vi "Resolve.vi"(8 "error in (no error)":errorcluster, 10 "Result (None)":refnum<class>, 11 "Promise in":refnum<class "Promise.lvclass">) -> (0 "error out":errorcluster, 3 "Promise out":refnum<class "Promise.lvclass">)   [LabVIEW 2020, in "Promises.lvlib" / "Promise.lvclass"]
doc: "<b>THIS VI DOES NOT PROPAGATE ERRORS</b>\nThis VI will generate an error if the Promise has already been resolved or is otherwise invalid.\n\nResolves the Promise with the provided Result value unless an error is passed in which will be encapsulated into the response and sent to the Future to return."
uses:
  Promise.lvclass
  Promise.lvclass/Promise.ctl
  Result.ctl
  Result State.ctl
  Error Result/Error Result.lvclass/Error Result.ctl
  Variant/Variant.lvclass
  Error Result/Error Result.lvclass
  Promises.lvlib
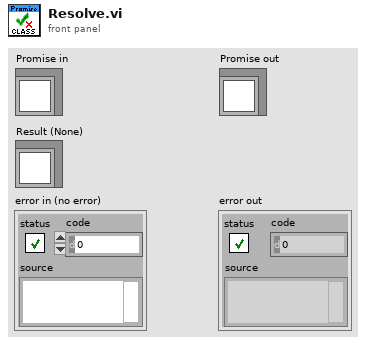
[diagram p1: front panel]
types:
  T1 = typedef "Promises.lvlib/Result.ctl" = cluster{"State":T2, "Value":refnum<class>}
  T2 = typedef "Promises.lvlib/Result State.ctl" = enum16{"Unset", "Error", "Success"}
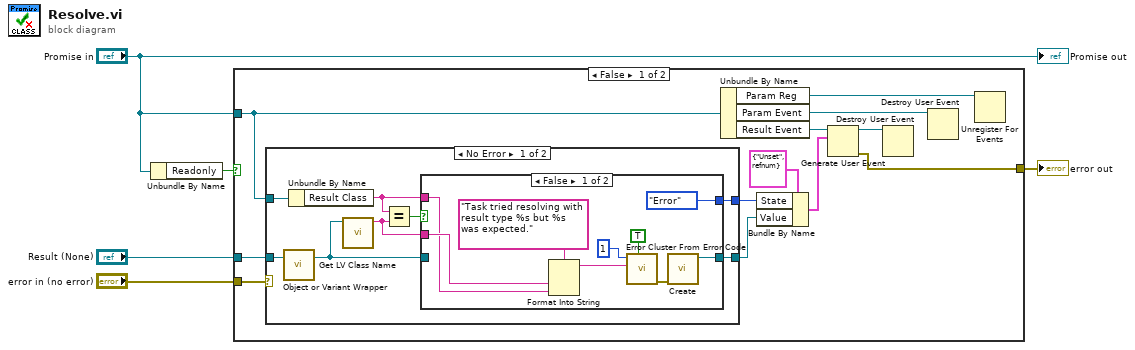
[diagram p0: block diagram]
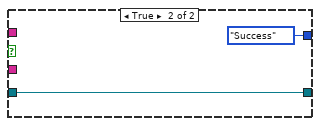
[diagram p2: hidden frame]
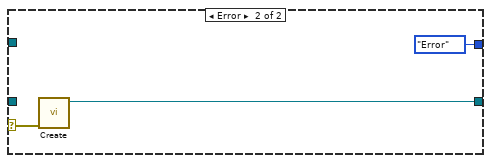
[diagram p3: hidden frame]
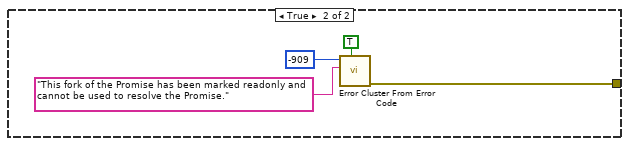
[diagram p4: hidden frame]
diagram:
  n1 = Unbundle By Name("Promise in") -> ("Readonly"=w1:bool)
  n2 = case shown="False" w1 {
    tunnel: "error in (no error)" -> [w17 _]
    tunnel: "Result (None)" -> [w16 _]
    tunnel: [w9 w43] -> w3
    tunnel: "Promise in" -> [w8 _]
    frame False {
      n3 = case shown="No Error" w17 {
        selector: w17 -> [_ w39]
        tunnel: w16 -> [w24 _]
        tunnel: [w20 w38] -> w13
        tunnel: w8 -> [w25 _]
        tunnel: [w19 Result_State."Error" ("Result State")] -> w14
        frame No Error {
          n4 = call "Object or Variant Wrapper.vi"("LabVIEW Object"=w24) -> ("Object or Variant Wrapper"=w18:refnum<class>)  [unwired: 6 in]
          n5 = Unbundle By Name(w25) -> ("Result Class"=w22:string)
          n6 = call <vilib>:"Get LV Class Name.vi"("object"=w18) -> ("class name"=w21:string)  [unwired: 9 in, 1 out]
          n7 = Equal?(x=w22, y=w21) -> (x = y?=w23:bool)
          n8 = case shown="False" w23 {
            tunnel: w18 -> [_ w36]
            tunnel: w22 -> [w33 _]
            tunnel: w21 -> [w34 _]
            tunnel: [w27 w36] -> w20
            tunnel: [Result_State."Error" ("Result State") Result_State."Success" ("Result State")] -> w19
            frame False {
              n9 = Format Into String(format string="Task tried resolving with result type %s but %s was expected.", w34, w33) -> (resulting string=w31:string)  [unwired: 2 in, 1 out]
              n10 = call <vilib>:"Error Cluster From Error Code.vi"("show call chain? (False)"=TRUE, "error message (\"\")"=w31, "error code (0)"=1) -> ("error out"=w28:errorcluster)  [unwired: 6 in]
              n11 = call "Create.vi"("error in (no error)"=w28) -> ("Error Result out"=w27:refnum<class "Error Result.lvclass">)  [unwired: 9 in, 1 out]
            }
            frame True {
            }
          }
        }
        frame Error {
          n12 = call "Create.vi"("error in (no error)"=w39) -> ("Error Result out"=w38:refnum<class "Error Result.lvclass">)  [unwired: 9 in, 1 out]
        }
      }
      n13 = Unbundle By Name(w8) -> ("Param Reg"=w6:refnum<event-registration>, "Param Event"=w7:refnum<user-event>, "Result Event"=w15:refnum<user-event>)
      n14 = Bundle By Name(cluster=T1 {"State"=enum."Unset", "Value"=refnum} ("event data"), "State"=w14, "Value"=w13) -> (w11:T1)
      n15 = Generate User Event(user event=w15, event data cluster=w11) -> (user event out=w10:refnum<user-event>, error out=w9:errorcluster)  [unwired: 2 in]
      n16 = Destroy User Event(user event=w10) -> ()  [unwired: 1 in, 1 out]
      n17 = Destroy User Event(user event=w7) -> ()  [unwired: 1 in, 1 out]
      n18 = Unregister For Events(event registration refnum=w6) -> ()  [unwired: 1 in, 1 out]
    }
    frame True {
      n19 = call <vilib>:"Error Cluster From Error Code.vi"("show call chain? (False)"=TRUE, "error message (\"\")"="This fork of the Promise has been marked readonly and cannot be used to resolve the Promise.", "error code (0)"=-909) -> ("error out"=w43:errorcluster)  [unwired: 6 in]
    }
  }
  "error out" <- w3
  "Promise out" <- "Promise in"
